vi "Tosca-Plot Histogram.vi"(0 "Histogram":refnum<vi>, 7 "Results":T1[](array[typedef]), 11 "error in (no error)":errorcluster) -> (15 "error out":errorcluster)   [LabVIEW 2020]
uses:
  Classes/Parameters/Histogram Data.ctl
  Classes/Parameters/Parameters.lvclass
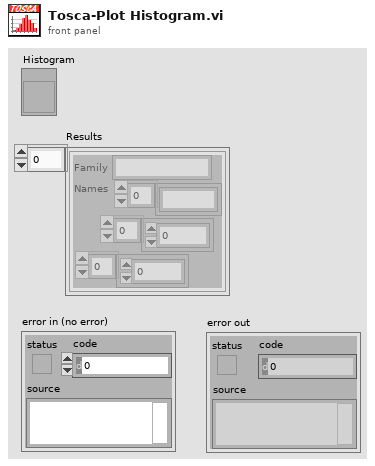
[diagram p1: front panel]
types:
  T1 = typedef "Parameters.lvclass/Histogram Data.ctl" = cluster{"Family":string, "Names":string[], "Colors":u32[], "N":i32[]}
  T2 = typedef "LVAnnotationListTypeDef.ctl" = cluster{"Name":string, "Color":u32, "Style":u8, "Point Style":u8, "Name Visible":bool, "Allow Drag":bool, "Annotation Mode":u32, "Plot":i32, "Index":i32, "Position":cluster{"X":dbl, "Y":dbl}, "X Scale":u32, "Y Scale":u32, "Show Arrow":bool, "Lock Name":bool, "Plot Area":i32, "Label Offset":cluster{"X":dbl, "Y":dbl}}[]
  T3 = cluster{"Name":string, "Color":u32, "Style":u8, "Point Style":u8, "Name Visible":bool, "Allow Drag":bool, "Annotation Mode":u32, "Plot":i32, "Index":i32, "Position":cluster{"X":dbl, "Y":dbl}, "X Scale":u32, "Y Scale":u32, "Show Arrow":bool, "Lock Name":bool, "Plot Area":i32, "Label Offset":cluster{"X":dbl, "Y":dbl}}
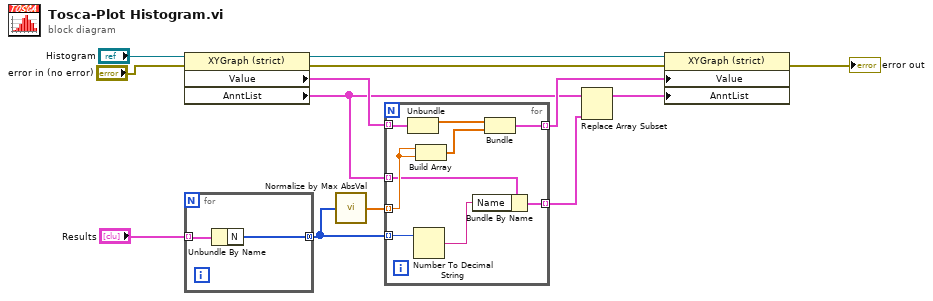
[diagram p0: block diagram]
diagram:
  n1 = property class="XYGraph (strict)"(reference="Histogram", error in="error in (no error)") -> (reference out=w8:refnum<vi>, error out=w7:errorcluster, "Value"=w10:cluster{dbl[], dbl[]}[], "AnntList"=w3:T2)
  n2 = for {
    tunnel: "Results" -> [w15] mode=indexing
    tunnel: [w14] -> w5 mode=concatenating
    n3 = Unbundle By Name(w15) -> ("N"=w14:i32[])
  }
  n4 = call "Normalize by Max AbsVal.vi"("Y"=w5) -> ("Ynorm"=w9:dbl[])
  n5 = for {
    tunnel: w10 -> [w24] mode=indexing
    tunnel: w3 -> [w19] mode=indexing
    tunnel: w9 -> [w22] mode=indexing
    tunnel: [w20] -> w6 mode=indexing
    tunnel: w5 -> [w18] mode=indexing
    tunnel: [w16] -> w2 mode=indexing
    n6 = Unbundle(w24) -> (w23:dbl[])  [unwired: 1 out]
    n7 = Number To Decimal String(number=w18) -> (decimal integer string=w17:string)  [unwired: 1 in]
    n8 = Build Array(w22, w22) -> (w21:dbl[])
    n9 = Bundle By Name(cluster=w19, "Name"=w17) -> (w16:T3)
    n10 = Bundle(w23, w21) -> (w20:cluster{dbl[], dbl[]})  [unwired: 1 in]
  }
  n11 = Replace Array Subset(array=w3, new element=w2) -> (w1:T2)  [unwired: 1 in]
  n12 = property class="XYGraph (strict)"(reference=w8, error in=w7, "Value"=w6, "AnntList"=w1) -> (error out=→"error out":errorcluster)  [unwired: 1 out]
